vi "HP4284A_CommandsGlobal.vi"() -> ()   [LabVIEW 2018, in "HP4284.lvclass"]
uses:
  HP4284.lvclass
panel:
  in  "HP 4284A GPIB Setup":T1={"Instrument name"="HP 4284A", "Instrument type"=1, "Command \"Initialise LCR\""=":FREQ %dHZ;:VOLT %fV;:FUNC:IMP:RANG:AUTO ON;:DISP:PAGE MEAS;:INIT:CONT OFF;:TRIG:SOUR HOLD", "Command \"OC Trim\""="CORR:OPEN:STATE ON", "Command \"LCR Readout\""="TRIG:DEL 0.0;:APER LONG,1;:TRIG:IMM;:FETC?"} {"Instrument type" items=["Supply", "LCR"]}
  # "Correction needs to be done manually.\nIt takes too long."
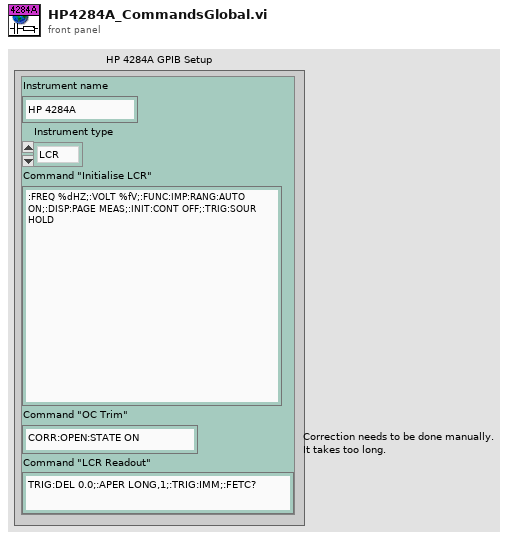
[diagram p1: front panel]
types:
  T1 = cluster{"Instrument name":string, "Instrument type":u16, "Command \"Initialise LCR\"":string, "Command \"OC Trim\"":string, "Command \"LCR Readout\"":string}
diagram:
